vi "Cluster Typedef JSON Staging.vi"(8 "error in (no error)":errorcluster) -> (0 "error out":errorcluster, 1 "Experiment Description 2":T1, 2 "JSON String":string)   [LabVIEW 2019]
uses:
  <vilib>/addons/_JKI.lib/Serialization/JSON/JKI JSON Serialization.lvlib
  Program Files (x86)/National Instruments/LabVIEW 2020/user.lib/LevyLab/Lockin-Multichannel/LockinDAQ/Typedefs/AO-cluster.ctl
  Program Files (x86)/National Instruments/LabVIEW 2020/user.lib/LevyLab/Lockin-Multichannel/LockinDAQ/LockinDAQ.lvclass
  Program Files (x86)/National Instruments/LabVIEW 2020/user.lib/LevyLab/Lockin-Multichannel/LockinDAQ/Typedefs/REF-cluster.ctl
  Program Files (x86)/National Instruments/LabVIEW 2020/user.lib/LevyLab/Lockin-Multichannel/LockinDAQ/Typedefs/Function-enum.ctl
  Program Files (x86)/National Instruments/LabVIEW 2020/user.lib/LevyLab/Krohn Hite 7008/typedefs/Channel-Enum.ctl
  Program Files (x86)/National Instruments/LabVIEW 2020/user.lib/LevyLab/Krohn Hite 7008/Instrument.KH7008.lvclass
  Program Files (x86)/National Instruments/LabVIEW 2020/user.lib/LevyLab/Krohn Hite 7008/typedefs/Gain-Enum.ctl
  Program Files (x86)/National Instruments/LabVIEW 2020/user.lib/LevyLab/Krohn Hite 7008/typedefs/Filter-Enum.ctl
  Program Files (x86)/National Instruments/LabVIEW 2020/user.lib/LevyLab/Krohn Hite 7008/typedefs/Shunt-Enum.ctl
  Program Files (x86)/National Instruments/LabVIEW 2020/user.lib/LevyLab/Krohn Hite 7008/typedefs/Coupling-Enum.ctl
  Program Files (x86)/National Instruments/LabVIEW 2020/user.lib/LevyLab/Krohn Hite 7008/typedefs/Input Configuration-Enum.ctl
  Program Files (x86)/National Instruments/LabVIEW 2020/user.lib/LevyLab/Krohn Hite 7008/typedefs/SetAll-Cluster.ctl
  Program Files (x86)/National Instruments/LabVIEW 2020/user.lib/LevyLab/Krohn Hite 7008/typedefs/SetAll-Array.ctl
panel:
  out "x = y?":T2
  out "from JSON (ms)":u32
  out "to JSON (ms)":u32
  in  "Experiment Description":T1
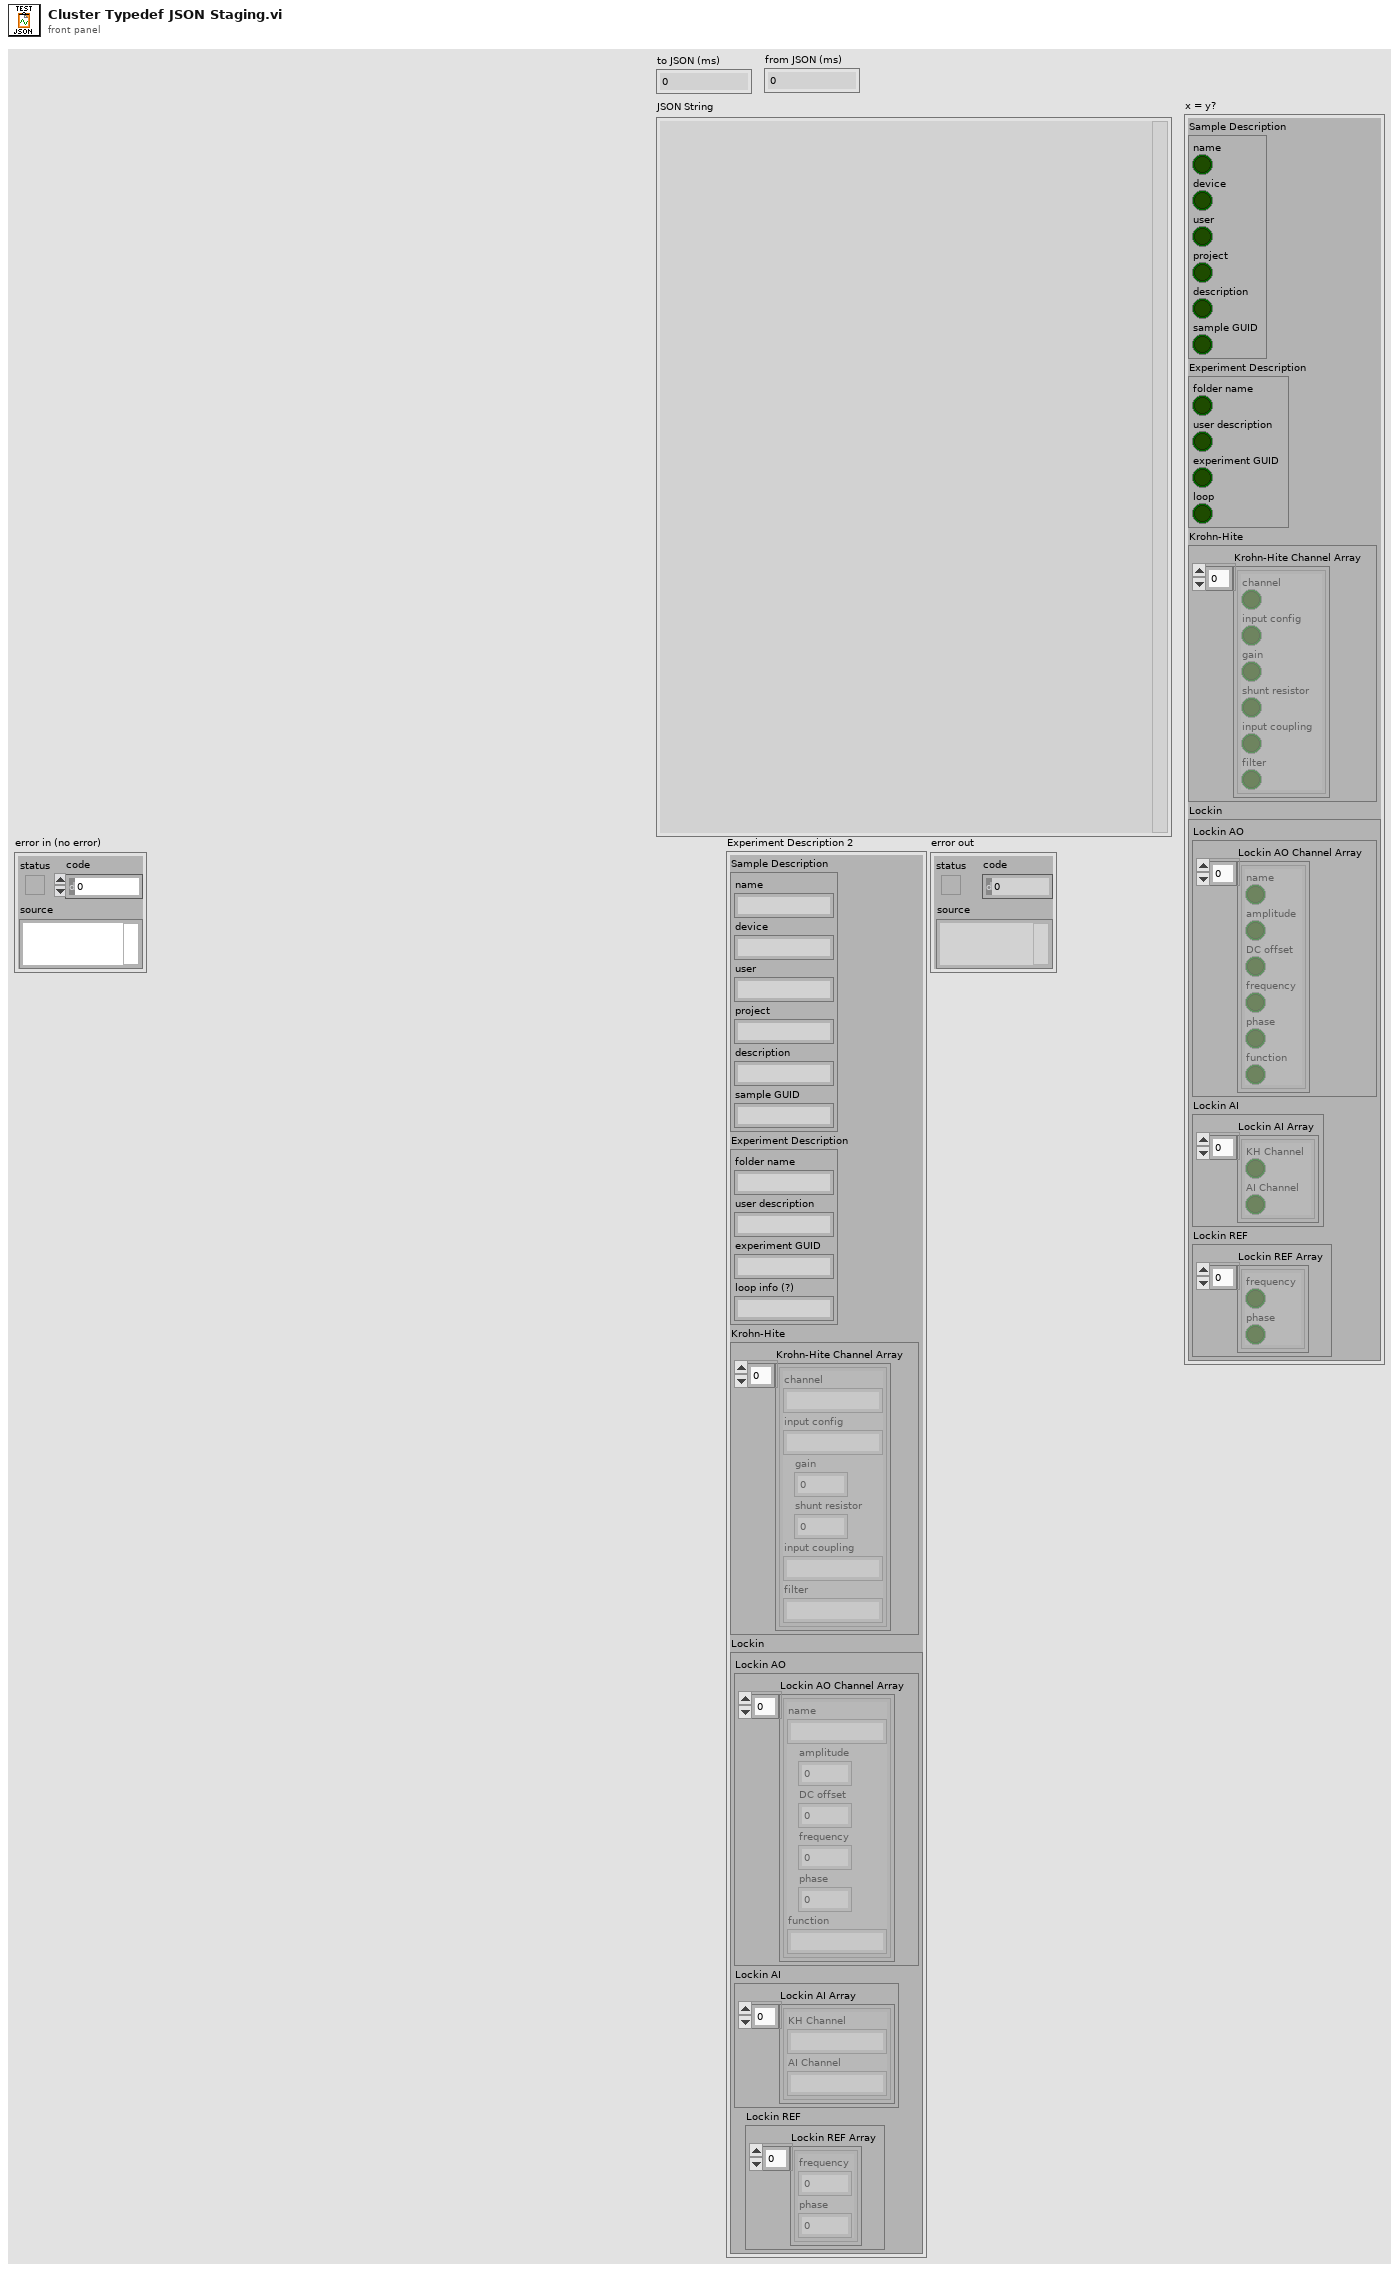
[diagram p1: front panel]
types:
  T1 = cluster{"Sample Description":cluster{"name":string, "device":string, "user":string, "project":string, "description":string, "sample GUID":string}, "Experiment Description":cluster{"folder name":string, "user description":string, "experiment GUID":string, "loop info (?)":string}, "Krohn-Hite":cluster{"Krohn-Hite Channel Array":cluster{"channel":string, "input config":string, "gain":i32, "shunt resistor":i32, "input coupling":string, "filter":string}[]}, "Lockin":cluster{"Lockin AO":cluster{"Lockin AO Channel Array":cluster{"name":string, "amplitude":dbl, "DC offset":dbl, "frequency":dbl, "phase":dbl, "function":string}[]}, "Lockin AI":cluster{"Lockin AI Array":cluster{"KH Channel":string, "AI Channel":string}[]}, "Lockin REF":cluster{"Lockin REF Array":cluster{"frequency":dbl, "phase":dbl}[]}}}
  T2 = cluster{"Sample Description":cluster{"name":bool, "device":bool, "user":bool, "project":bool, "description":bool, "sample GUID":bool}, "Experiment Description":cluster{"folder name":bool, "user description":bool, "experiment GUID":bool, "loop":bool}, "Krohn-Hite":cluster{"Krohn-Hite Channel Array":cluster{"channel":bool, "input config":bool, "gain":bool, "shunt resistor":bool, "input coupling":bool, "filter":bool}[]}, "Lockin":cluster{"Lockin AO":cluster{"Lockin AO Channel Array":cluster{"name":bool, "amplitude":bool, "DC offset":bool, "frequency":bool, "phase":bool, "function":bool}[]}, "Lockin AI":cluster{"Lockin AI Array":cluster{"KH Channel":bool, "AI Channel":bool}[]}, "Lockin REF":cluster{"Lockin REF Array":cluster{"frequency":bool, "phase":bool}[]}}}
  T3 = typedef "LockinDAQ.lvclass/REF-cluster.ctl" = cluster{"Ch":i32[], " f (Hz)":dbl[], "Phase (°)":dbl[], "TC (s)":dbl[], "order":i32[]}
  T4 = typedef "Instrument.KH7008.lvclass/SetAll-Array.ctl" = T5[]
  T5 = typedef "Instrument.KH7008.lvclass/SetAll-Cluster.ctl" = cluster{"Channel":T6, "Gain":T7, "Bandwidth Filter":T8, "Shunt Resistor":T9, "Coupling":T10, "Input Config":T11}
  T6 = typedef "Instrument.KH7008.lvclass/Channel-Enum.ctl" = enum16{"Channel 1", "Channel 2", "Channel 3", "Channel 4", "Channel 5", "Channel 6", "Channel 7", "Channel 8"}
  T7 = typedef "Instrument.KH7008.lvclass/Gain-Enum.ctl" = enum16{"1x", "10x", "100x", "1000x"}
  T8 = typedef "Instrument.KH7008.lvclass/Filter-Enum.ctl" = enum16{"OFF", "ON"}
  T9 = typedef "Instrument.KH7008.lvclass/Shunt-Enum.ctl" = enum16{"Open", "50 Ohms", "500 Ohms", "5k Ohms", "50k Ohms"}
  T10 = typedef "Instrument.KH7008.lvclass/Coupling-Enum.ctl" = enum16{"AC", "DC"}
  T11 = typedef "Instrument.KH7008.lvclass/Input Configuration-Enum.ctl" = enum16{"Ground", "SE+ (-gnd)", "SE- (+gnd)", "Differential"}
  T12 = typedef "LockinDAQ.lvclass/AO-cluster.ctl" = cluster{"Ch":i32[], "Amp (V)":dbl[], "DC (V)":dbl[], "f (Hz)":dbl[], "Phase (°)":dbl[], "Function":T13[], "Sweep?":bool[]}
  T13 = typedef "LockinDAQ.lvclass/Function-enum.ctl" = enum16{"Sine", "Triangle", "Square", "Sawtooth"}
  T14 = cluster{"name":string, "device":string, "user":string, "project":string, "description":string, "sample GUID":string}
  T15 = cluster{"folder name":string, "user description":string, "experiment GUID":string, "loop info (?)":string}
  T16 = cluster{"Krohn-Hite Channel Array":cluster{"channel":string, "input config":string, "gain":i32, "shunt resistor":i32, "input coupling":string, "filter":string}[]}
  T17 = cluster{"Lockin AO":cluster{"Lockin AO Channel Array":cluster{"name":string, "amplitude":dbl, "DC offset":dbl, "frequency":dbl, "phase":dbl, "function":string}[]}, "Lockin AI":cluster{"Lockin AI Array":cluster{"KH Channel":string, "AI Channel":string}[]}, "Lockin REF":cluster{"Lockin REF Array":cluster{"frequency":dbl, "phase":dbl}[]}}
  T18 = cluster{"Lockin AO Channel Array":cluster{"name":string, "amplitude":dbl, "DC offset":dbl, "frequency":dbl, "phase":dbl, "function":string}[]}
  T19 = cluster{"Lockin REF Array":cluster{"frequency":dbl, "phase":dbl}[]}
  T20 = cluster{"Lockin AI Array":cluster{"KH Channel":string, "AI Channel":string}[]}
  T21 = cluster{"channel":string, "input config":string, "gain":i32, "shunt resistor":i32, "input coupling":string, "filter":string}[]
  T22 = cluster{"channel":string, "input config":string, "gain":i32, "shunt resistor":i32, "input coupling":string, "filter":string}
  T23 = cluster{"name":string, "amplitude":dbl, "DC offset":dbl, "frequency":dbl, "phase":dbl, "function":string}[]
  T24 = cluster{"name":string, "amplitude":dbl, "DC offset":dbl, "frequency":dbl, "phase":dbl, "function":string}
  T25 = cluster{"KH Channel":string, "AI Channel":string}[]
  T26 = cluster{"KH Channel":string, "AI Channel":string}
  T27 = cluster{"Sample Description":cluster{"name":bool, "device":bool, "user":bool, "project":bool, "description":bool, "sample GUID":bool}, "Experiment Description":cluster{"folder name":bool, "user description":bool, "experiment GUID":bool, "loop info (?)":bool}, "Krohn-Hite":cluster{"Krohn-Hite Channel Array":cluster{"channel":bool, "input config":bool, "gain":bool, "shunt resistor":bool, "input coupling":bool, "filter":bool}[]}, "Lockin":cluster{"Lockin AO":cluster{"Lockin AO Channel Array":cluster{"name":bool, "amplitude":bool, "DC offset":bool, "frequency":bool, "phase":bool, "function":bool}[]}, "Lockin AI":cluster{"Lockin AI Array":cluster{"KH Channel":bool, "AI Channel":bool}[]}, "Lockin REF":cluster{"Lockin REF Array":cluster{"frequency":bool, "phase":bool}[]}}}
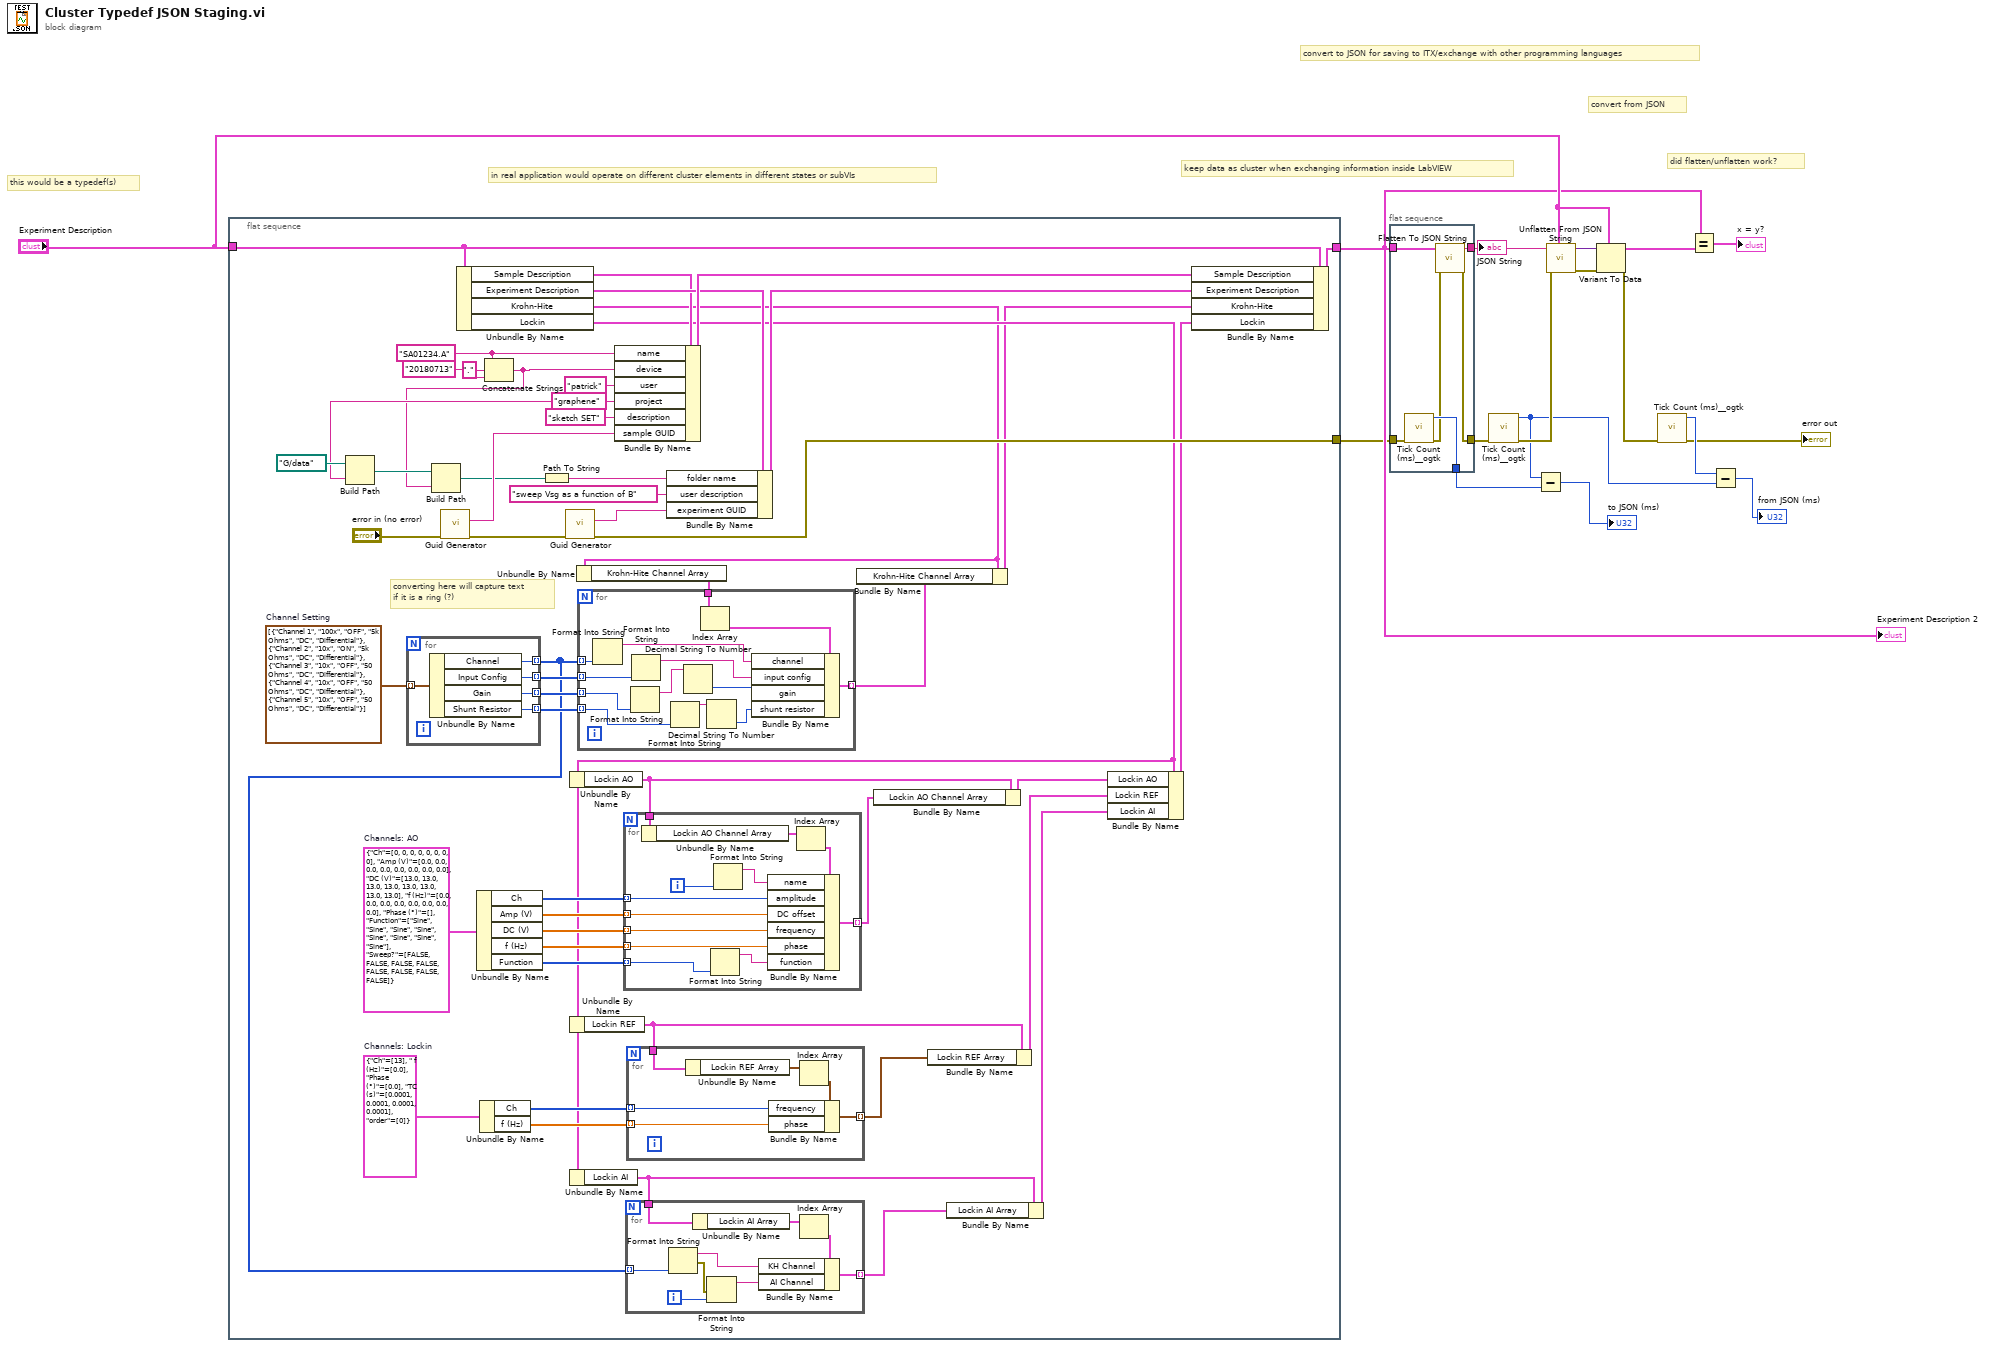
[diagram p0: block diagram]
diagram:
  # "keep data as cluster when exchanging information inside LabVIEW"
  # "did flatten/unflatten work?"
  # "convert from JSON"
  # "convert to JSON for saving to ITX/exchange with other programming languages"
  # "in real application would operate on different cluster elements in different states or subVIs"
  # "this would be a typedef(s)"
  n1 = flat-sequence {
    tunnel: "Experiment Description" -> [w33]
    tunnel: [w32] -> w3
    tunnel: [w24] -> w2
    frame #0 {
      w42 = T3 {"Ch"=[13], " f (Hz)"=[0.0], "Phase (°)"=[0.0], "TC (s)"=[0.0001, 0.0001, 0.0001, 0.0001], "order"=[0]}  # Channels: Lockin
      w48 = "SA01234.A" ("name")
      w35 = "graphene" ("project")
      w68 = T4 [{"Channel"=enum."Channel 1", "Gain"=enum."100x", "Bandwidth Filter"=enum."OFF", "Shunt Resistor"=enum."5k Ohms", "Coupling"=enum."DC", "Input Config"=enum."Differential"}, {"Channel"=enum."Channel 2", "Gain"=enum."10x", "Bandwidth Filter"=enum."ON", "Shunt Resistor"=enum."5k Ohms", "Coupling"=enum."DC", "Input Config"=enum."Differential"}, {"Channel"=enum."Channel 3", "Gain"=enum."10x", "Bandwidth Filter"=enum."OFF", "Shunt Resistor"=enum."50 Ohms", "Coupling"=enum."DC", "Input Config"=enum."Differential"}, {"Channel"=enum."Channel 4", "Gain"=enum."10x", "Bandwidth Filter"=enum."OFF", "Shunt Resistor"=enum."50 Ohms", "Coupling"=enum."DC", "Input Config"=enum."Differential"}, {"Channel"=enum."Channel 5", "Gain"=enum."10x", "Bandwidth Filter"=enum."OFF", "Shunt Resistor"=enum."50 Ohms", "Coupling"=enum."DC", "Input Config"=enum."Differential"}]  # Channel Setting
      w61 = T12 {"Ch"=[0, 0, 0, 0, 0, 0, 0, 0], "Amp (V)"=[0.0, 0.0, 0.0, 0.0, 0.0, 0.0, 0.0, 0.0], "DC (V)"=[13.0, 13.0, 13.0, 13.0, 13.0, 13.0, 13.0, 13.0], "f (Hz)"=[0.0, 0.0, 0.0, 0.0, 0.0, 0.0, 0.0, 0.0], "Phase (°)"=[], "Function"=[enum."Sine", enum."Sine", enum."Sine", enum."Sine", enum."Sine", enum."Sine", enum."Sine", enum."Sine"], "Sweep?"=[FALSE, FALSE, FALSE, FALSE, FALSE, FALSE, FALSE, FALSE]}  # Channels: AO
      # "converting here will capture text\nif it is a ring (?)"
      n2 = Build Path(base path=path "G:/data", name or relative path=w35) -> (appended path=w45:path)
      n3 = for {
        tunnel: w68 -> [w101] mode=indexing
        tunnel: [w100] -> w28 mode=indexing
        tunnel: [w99] -> w67 mode=indexing
        tunnel: [w98] -> w66 mode=indexing
        tunnel: [w97] -> w65 mode=indexing
        n4 = Unbundle By Name(w101) -> ("Channel"=w100:T6, "Input Config"=w99:T11, "Gain"=w98:T7, "Shunt Resistor"=w97:T9)
      }
      n5 = call <vilib>:"Guid Generator.vi"("error in (no error)"="error in (no error)") -> ("error out"=w23:errorcluster, "GUID"=w46:string)  [unwired: 9 in]
      n6 = Unbundle By Name(w33) -> ("Sample Description"=w29:T14, "Experiment Description"=w30:T15, "Krohn-Hite"=w20:T16, "Lockin"=w21:T17)
      n7 = Unbundle By Name(w61) -> ("Ch"=w60:i32[], "Amp (V)"=w59:dbl[], "DC (V)"=w57:dbl[], "f (Hz)"=w56:dbl[], "Function"=w55:T13[])
      n8 = Unbundle By Name(w42) -> ("Ch"=w41:i32[], "f (Hz)"=w40:dbl[])
      n9 = Concatenate Strings(w48, "." ("string"), "20180713" ("device")) -> (w34:string)
      n10 = Build Path(base path=w45, name or relative path=w34) -> (appended path=w44:path)
      n11 = Path To String(path=w44) -> (string=w43:string)
      n12 = call <vilib>:"Guid Generator.vi"("error in (no error)"=w23) -> ("error out"=w24:errorcluster, "GUID"=w54:string)  [unwired: 9 in]
      n13 = Unbundle By Name(w21) -> ("Lockin AO"=w31:T18)
      n14 = Unbundle By Name(w21) -> ("Lockin REF"=w39:T19)
      n15 = Unbundle By Name(w21) -> ("Lockin AI"=w37:T20)
      n16 = Unbundle By Name(w20) -> ("Krohn-Hite Channel Array"=w63:T21)
      n17 = for {
        tunnel: w63 -> [w111]
        tunnel: [w114] -> w62 mode=indexing
        tunnel: w28 -> [w113] mode=indexing
        tunnel: w67 -> [w112] mode=indexing
        tunnel: w66 -> [w107] mode=indexing
        tunnel: w65 -> [w106] mode=indexing
        n18 = Format Into String(w113) -> (resulting string=w108:string)  [unwired: 3 in, 1 out]
        n19 = Format Into String(w107) -> (resulting string=w104:string)  [unwired: 3 in, 1 out]
        n20 = Format Into String(w112) -> (resulting string=w109:string)  [unwired: 3 in, 1 out]
        n21 = Format Into String(w106) -> (resulting string=w105:string)  [unwired: 3 in, 1 out]
        n22 = Decimal String To Number(string=w104) -> (number=w103:i32)  [unwired: 2 in, 1 out]
        n23 = Index Array(array=w111) -> (element=w110:T22)  [unwired: 1 in]
        n24 = Decimal String To Number(string=w105) -> (number=w102:i32)  [unwired: 2 in, 1 out]
        n25 = Bundle By Name(cluster=w110, "channel"=w108, "input config"=w109, "gain"=w103, "shunt resistor"=w102) -> (w114:T22)
      }
      n26 = Bundle By Name(cluster=w29, "name"=w48, "device"=w34, "user"="patrick", "project"=w35, "description"="sketch SET", "sample GUID"=w46) -> (w64:T14)
      n27 = for {
        tunnel: w31 -> [w92]
        tunnel: [w96] -> w27 mode=indexing
        tunnel: w60 -> [w94] mode=indexing
        tunnel: w59 -> [w93] mode=indexing
        tunnel: w57 -> [w90] mode=indexing
        tunnel: w56 -> [w89] mode=indexing
        tunnel: w55 -> [w88] mode=indexing
        i -> [w95]
        n28 = Unbundle By Name(w92) -> ("Lockin AO Channel Array"=w91:T23)
        n29 = Format Into String(w88) -> (resulting string=w86:string)  [unwired: 3 in, 1 out]
        n30 = Format Into String(w95) -> (resulting string=w87:string)  [unwired: 3 in, 1 out]
        n31 = Index Array(array=w91) -> (element=w85:T24)  [unwired: 1 in]
        n32 = Bundle By Name(cluster=w85, "name"=w87, "amplitude"=w94, "DC offset"=w93, "frequency"=w90, "phase"=w89, "function"=w86) -> (w96:T24)
      }
      n33 = for {
        tunnel: w37 -> [w73]
        tunnel: [w78] -> w25 mode=indexing
        tunnel: w28 -> [w75] mode=indexing
        i -> [w76]
        n34 = Format Into String(w75) -> (resulting string=w74:string, error out=w70:errorcluster)  [unwired: 3 in]
        n35 = Unbundle By Name(w73) -> ("Lockin AI Array"=w77:T25)
        n36 = Format Into String(error in=w70, w76) -> (resulting string=w71:string)  [unwired: 2 in, 1 out]
        n37 = Index Array(array=w77) -> (element=w72:T26)  [unwired: 1 in]
        n38 = Bundle By Name(cluster=w72, "KH Channel"=w74, "AI Channel"=w71) -> (w78:T26)
      }
      n39 = for {
        tunnel: w39 -> [w80]
        tunnel: [w84] -> w26 mode=indexing
        tunnel: w41 -> [w82] mode=indexing
        tunnel: w40 -> [w81] mode=indexing
        n40 = Unbundle By Name(w80) -> ("Lockin REF Array"=w83:cluster{"frequency":dbl, "phase":dbl}[])
        n41 = Index Array(array=w83) -> (element=w79:cluster{"frequency":dbl, "phase":dbl})  [unwired: 1 in]
        n42 = Bundle By Name(cluster=w79, "frequency"=w82, "phase"=w81) -> (w84:cluster{"frequency":dbl, "phase":dbl})
      }
      n43 = Bundle By Name(cluster=w30, "folder name"=w43, "user description"="sweep Vsg as a function of B" ("description"), "experiment GUID"=w54) -> (w69:T15)
      n44 = Bundle By Name(cluster=w20, "Krohn-Hite Channel Array"=w62) -> (w19:T16)
      n45 = Bundle By Name(cluster=w31, "Lockin AO Channel Array"=w27) -> (w58:T18)
      n46 = Bundle By Name(cluster=w39, "Lockin REF Array"=w26) -> (w38:T19)
      n47 = Bundle By Name(cluster=w37, "Lockin AI Array"=w25) -> (w36:T20)
      n48 = Bundle By Name(cluster=w21, "Lockin AO"=w58, "Lockin REF"=w38, "Lockin AI"=w36) -> (w18:T17)
      n49 = Bundle By Name(cluster=w33, "Sample Description"=w64, "Experiment Description"=w69, "Krohn-Hite"=w19, "Lockin"=w18) -> (w32:T1)
    }
  }
  n50 = flat-sequence {
    tunnel: [w120] -> w17
    tunnel: [w119] -> w14
    tunnel: w3 -> [w118]
    tunnel: [w117] -> w8
    tunnel: w2 -> [w115]
    frame #0 {
      n51 = call "Tick Count (ms)__ogtk.vi"("error in (no error)"=w115) -> ("error out"=w116:errorcluster, "millisecond timer value"=w117:u32)  [unwired: 9 in]
      n52 = call <vilib>:"Flatten To JSON String.vi"("error in (no error)"=w116, "Variant"=w118) -> ("error out"=w119:errorcluster, "JSON String"=w120:string)  [unwired: 8 in]
    }
  }
  n53 = call "Tick Count (ms)__ogtk.vi"("error in (no error)"=w14) -> ("error out"=w13:errorcluster, "millisecond timer value"=w6:u32)  [unwired: 9 in]
  n54 = Subtract(x=w6, y=w8) -> (x-y=→"to JSON (ms)":u32)
  n55 = call <vilib>:"Unflatten From JSON String.vi"("Type and Defaults"="Experiment Description", "error in (no error)"=w13, "JSON String"=w17) -> ("error out"=w16:errorcluster, "Variant"=w15:variant)  [unwired: 7 in]
  n56 = Variant To Data(error in=w16, type="Experiment Description", Variant=w15) -> (data=w9:T1, error out=w12:errorcluster)
  n57 = call "Tick Count (ms)__ogtk.vi"("error in (no error)"=w12) -> ("error out"=→"error out":errorcluster, "millisecond timer value"=w7:u32)  [unwired: 9 in]
  n58 = Equal?(x=w3, y=w9) -> (x = y?=→"x = y?":T27)
  n59 = Subtract(x=w7, y=w6) -> (x-y=→"from JSON (ms)":u32)
  "JSON String" <- w17
  "Experiment Description 2" <- w3
